vi "Example Polymorphic 2.vi"() -> ()   [LabVIEW 2014]
uses:
  Transcriptors/System API/Serial println string.vi
  Transcriptors/System API/Serial print string.vi
  Transcriptors/System API/Serial println integer.vi
  Transcriptors/System API/Serial print integer.vi
  Transcriptors/System API/Serial print frac number.vi
panel:
  out "Error Out":errorcluster
  in  "Error In":errorcluster
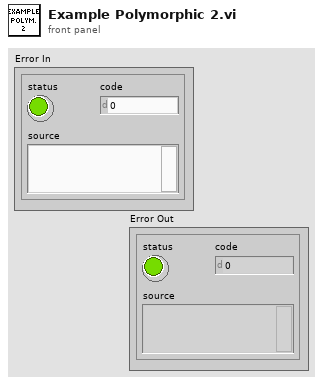
[diagram p1: front panel]
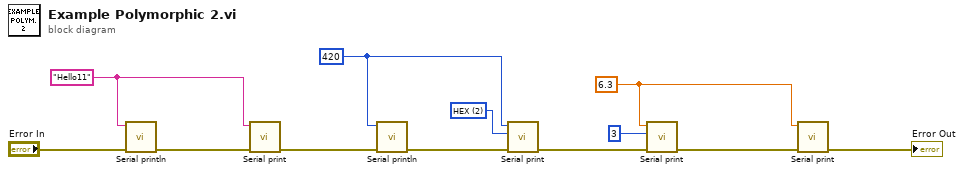
[diagram p0: block diagram]
diagram:
  w1 = 6.3 ("number in")
  w3 = u16 2 items=["BIN", "OCT", "HEX", "DEC"] ("format")
  w4 = 420 ("number to print")
  w5 = "Hello11" ("string in")
  n1 = call-poly "Serial println.vi"("Error In"="Error In", "string in"=w5) -> ("Error Out"=w11:errorcluster)  [unwired: 9 in]
  n2 = call-poly "Serial print.vi"("Error In"=w11, "string in"=w5) -> ("Error Out"=w10:errorcluster)  [unwired: 9 in]
  n3 = call-poly "Serial println.vi"("Error In"=w10, "number to print"=w4) -> ("Error Out"=w9:errorcluster)  [unwired: 9 in]
  n4 = call-poly "Serial print.vi"("Error In"=w9, "format"=w3, "number to print"=w4) -> ("Error Out"=w8:errorcluster)  [unwired: 8 in]
  n5 = call-poly "Serial print.vi"("Error In"=w8, "precision"=i16 3, "number in"=w1) -> ("Error Out"=w7:errorcluster)  [unwired: 8 in]
  n6 = call-poly "Serial print.vi"("Error In"=w7, "number in"=w1) -> ("Error Out"=→"Error Out":errorcluster)  [unwired: 9 in]
